vi "Build Name.vi"(0 "Pin":string, 9 "Site":string) -> (4 "Path name":string)   [LabVIEW 2023, in "RFCalAndFixtureCharact.Common.lvlib" / "Path.lvclass"]
uses:
  Path.lvclass
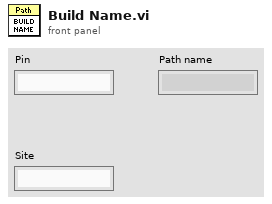
[diagram p1: front panel]
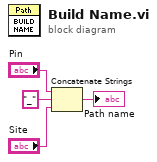
[diagram p0: block diagram]
diagram:
  n1 = Concatenate Strings("Pin", "_" ("string"), "Site") -> (→"Path name":string)
